vi "Load and split packets from file_old.vi"(8 "error in":errorcluster, 11 "Path":path) -> (0 "error out":errorcluster, 2 "OK?":bool, 3 "Hex Array":string[](array[string]))   [LabVIEW 2020]
panel:
  out "Normal Array":string[](array[string])
  out "selected path":path
  out "text":string
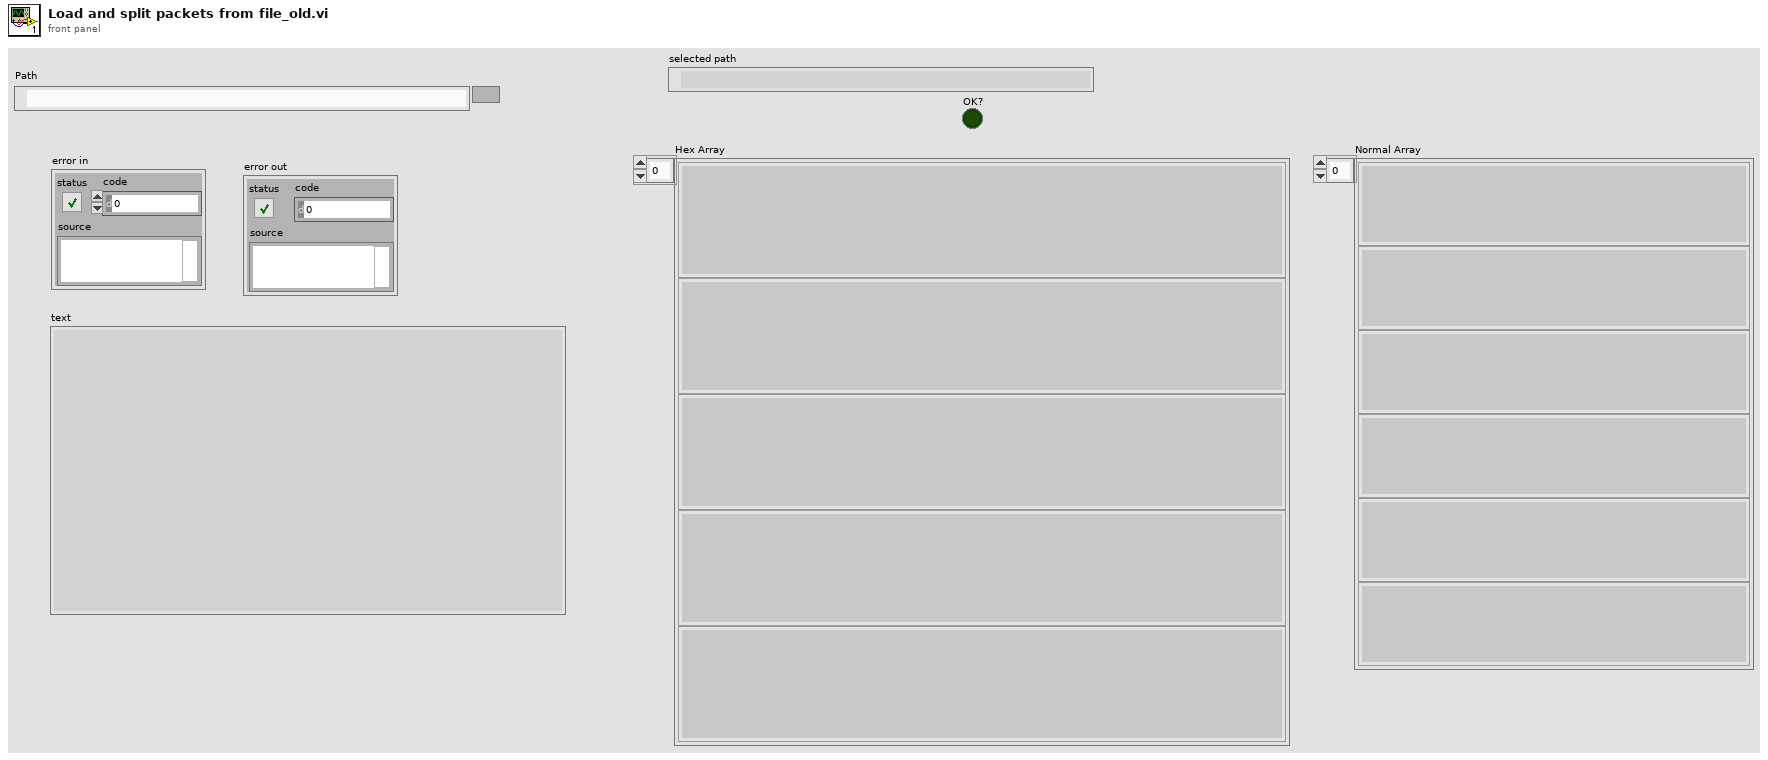
[diagram p1: front panel]
types:
  T1 = enum16{"open", "replace", "create", "open or create", "replace or create", "replace or create with confirmation"}
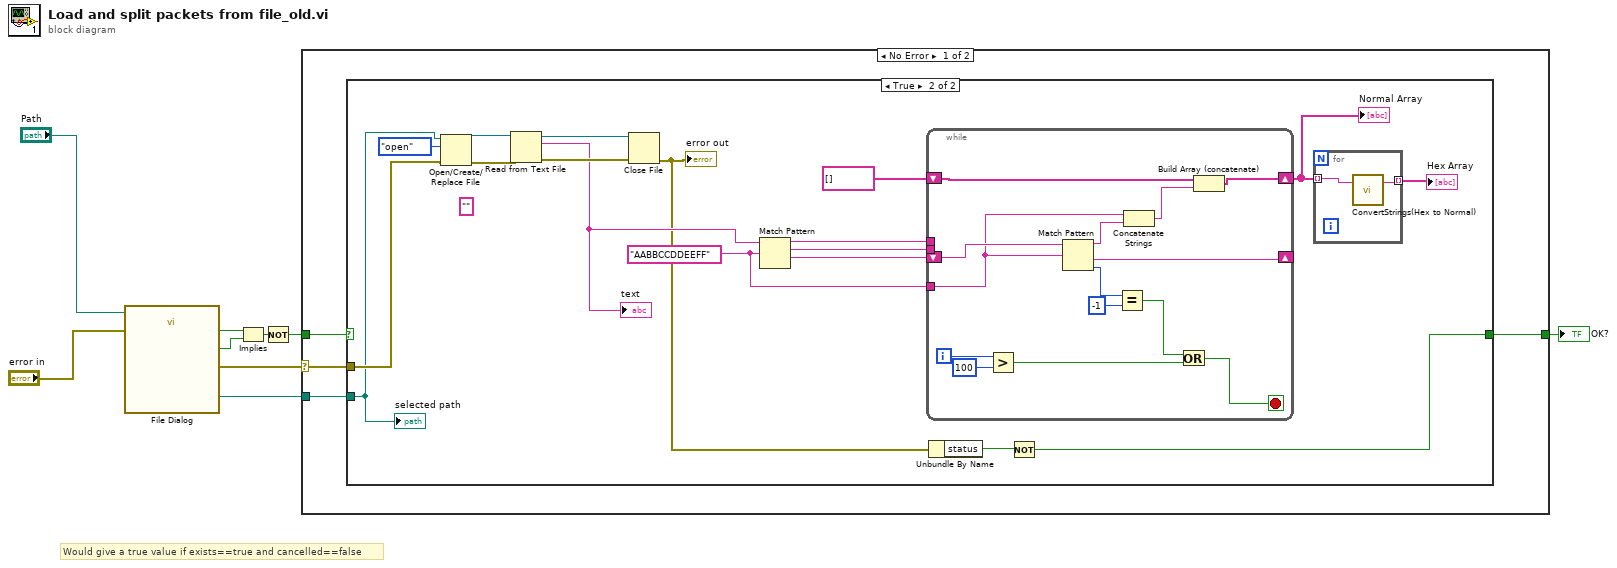
[diagram p0: block diagram]
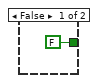
[diagram p2: hidden frame]
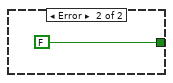
[diagram p3: hidden frame]
diagram:
  # "Would give a true value if exists==true and cancelled==false"
  n1 = call "File Dialog"("start path"="Path", "error in"="error in") -> ("selected path"=w2:path, "exists"=w5:bool, "cancelled"=w4:bool, "error out"=w7:errorcluster)  [unwired: 10 in]
  n2 = Implies(1:w4, 2:w5) -> (0:w6:bool)
  n3 = Not(x=w6) -> (.not. x?=w3:bool)
  n4 = case shown="No Error" w7 {
    selector: w7 -> [w12 _]
    tunnel: w3 -> [w13 _]
    tunnel: w2 -> [w11 _]
    tunnel: [w10 FALSE] -> w1
    frame No Error {
      n5 = case shown="True" w13 {
        tunnel: w12 -> [_ w23]
        tunnel: w11 -> [_ w22]
        tunnel: [FALSE w15] -> w10
        frame False {
        }
        frame True {
          (unwired) ""
          w24 = "AABBCCDDEEFF" ("regular expression")
          n6 = Open/Create/Replace File(file path (use dialog)=w22, error in=w23, operation (0:open)=T1."open") -> (refnum out=w30:refnum<file>, error out=w31:errorcluster)  [unwired: 3 in, 1 out]
          n7 = Read from Text File(file (use dialog)=w30, error in=w31) -> (refnum out=w28:refnum<file>, text=w21:string, error out=w29:errorcluster)  [unwired: 2 in, 1 out]
          "text" <- w21
          n8 = Close File(refnum=w28, error in=w29) -> (error out=w17:errorcluster)  [unwired: 1 out]
          "error out" <- w17
          n9 = Match Pattern(string=w21, regular expression=w24) -> (before substring=w27:string, match substring=w26:string, after substring=w25:string)  [unwired: 1 in, 1 out]
          n10 = while {
            tunnel: w27 -> [_]
            tunnel: w26 -> [_]
            shift-right: [w44] -> w19
            shift-left: string[] [] -> [w45]
            tunnel: w24 -> [w46]
            shift-right: [w42] -> _
            shift-left: w25 -> [w48]
            i -> [w39]
            stop <- w35 stop-if-true
            n11 = Greater?(x=w39, y=100) -> (0:w36:bool)
            n12 = Match Pattern(string=w48, regular expression=w46) -> (before substring=w47:string, after substring=w42:string, offset past match=w41:i32)  [unwired: 1 in, 1 out]
            n13 = Equal?(x=w41, y=-1) -> (x = y?=w37:bool)
            n14 = Concatenate Strings(w46, w47) -> (w43:string)
            n15 = Or(x=w37, y=w36) -> (x .or. y?=w35:bool)
            n16 = Build Array (concatenate)(w45, w43) -> (w44:string[])
          }
          "Normal Array" <- w19
          n17 = Unbundle By Name(w17) -> ("status"=w16:bool)
          n18 = Not(x=w16) -> (.not. x?=w15:bool)
          n19 = for {
            tunnel: w19 -> [w34] mode=indexing
            tunnel: [w33] -> w18 mode=indexing
            n20 = call "ConvertStrings(Hex to Normal).vi"("Hex String"=w34) -> ("Normal String"=w33:string)  [unwired: 2 in]
          }
          "Hex Array" <- w18
          "selected path" <- w22
        }
      }
    }
    frame Error {
    }
  }
  "OK?" <- w1
